vi "4bar encoder to angle.vi"(1 "Encoder Position":dbl) -> (0 "4bar Angle Radians":dbl)   [LabVIEW 2018]
uses:
  Infrastructure/Constants.vi
panel:
  in  "4bar Angle Degrees":dbl
  in  "4bar Angle Radians":dbl
  out "Encoder Position":dbl
  # "1 raw encoder count is .375 degrees"
  # "960 counts in 360 degrees"
  # "make 0 be horizantal"
  # "ratio might change ^^^"
  # "encoder count ---->  angle"
  # "angle ----> encoder count"
  # "(probably not needed)"
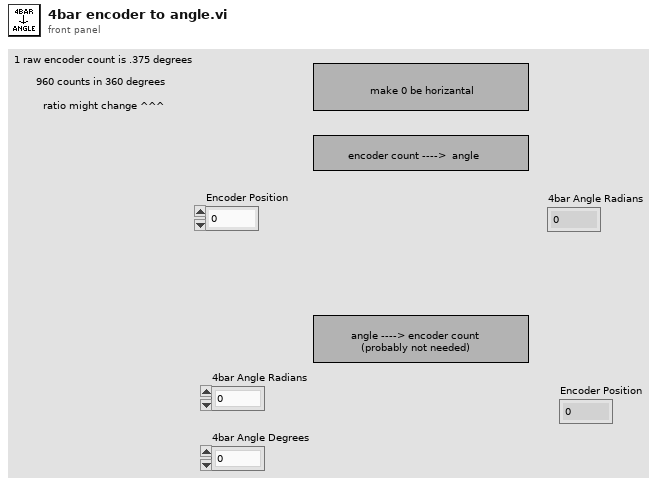
[diagram p1: front panel]
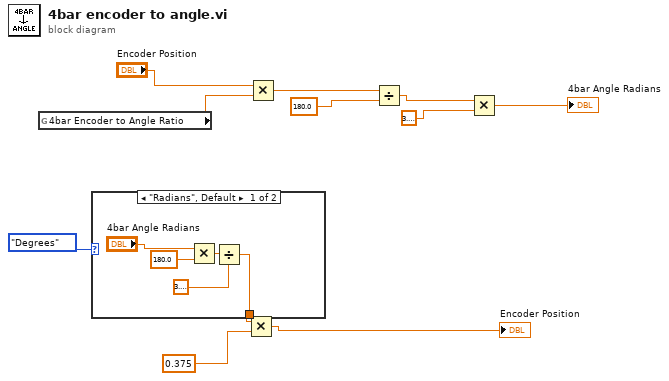
[diagram p0: block diagram]
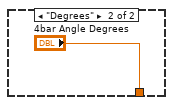
[diagram p2: hidden frame]
diagram:
  n1 = global read "Constants.vi" "4bar Encoder to Angle Ratio"() -> (w1:dbl)
  n2 = case shown="\"Radians\", Default" enum16{"Radians", "Degrees"}."Degrees" {
    tunnel: [w12 "4bar Angle Degrees"] -> w2
    frame "Radians", Default {
      n3 = Multiply(x="4bar Angle Radians", y=180.0) -> (x*y=w14:dbl)
      n4 = Divide(x=w14, y=3.141592653589793) -> (x/y=w12:dbl)
    }
    frame "Degrees" {
    }
  }
  n5 = Multiply(x=w2, y=0.375) -> (x*y=→"Encoder Position":dbl)
  n6 = Multiply(x="Encoder Position", y=w1) -> (x*y=w7:dbl)
  n7 = Divide(x=w7, y=180.0) -> (x/y=w6:dbl)
  n8 = Multiply(x=w6, y=3.141592653589793) -> (x*y=→"4bar Angle Radians":dbl)
